vi "AddPassed.vi"(8 "error in (no error)":errorcluster, 10 "TestCase":refnum<class "TestCase.lvclass">, 11 "TestResult in":refnum<class "TestResult.lvclass">) -> (0 "error out":errorcluster, 3 "TestResult out":refnum<class "TestResult.lvclass">)   [LabVIEW 2019, in "TestResult.lvclass"]
doc: "Adds a test to the list of passed tests."
uses:
  TestResult.lvclass
  TestCase/TestCase/TestCase.lvclass
  TestResult.lvclass/TestResult.ctl
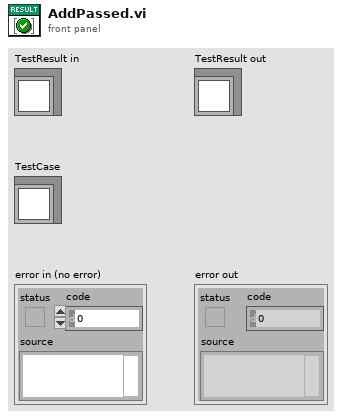
[diagram p1: front panel]
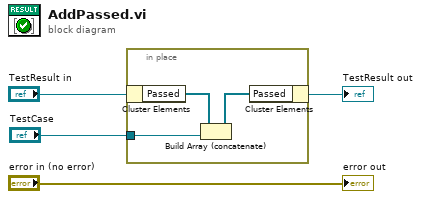
[diagram p0: block diagram]
diagram:
  n1 = in-place {
    in-place-border: "TestCase" -> [w5]
    n2 = in-place-cluster #1("TestResult in") -> ("Passed"=w7:refnum<class "TestCase.lvclass">[])
    n3 = Build Array (concatenate)(w7, w5) -> (w6:refnum<class "TestCase.lvclass">[])
    n4 = in-place-cluster #1("Passed"=w6) -> (→"TestResult out":refnum<class "TestResult.lvclass">)
  }
  "error out" <- "error in (no error)"
